vi "Update Enum Getter.vi"(7 "RPC Message Name":string, 8 "error in (no error)":errorcluster, 10 "Message Getter in":refnum<vi>, 11 "RPC Messages Folder (ProjectItem) in":refnum<vi>) -> (0 "error out":errorcluster, 2 "Message Getter out":refnum<vi>, 3 "RPC Messages Folder (ProjectItem) out":refnum<vi>)   [LabVIEW 2019, in "gRPC Template Creation Utility.lvlib"]
uses:
  gRPC Template Creation Utility.lvlib
  <vilib>/Utility/traverseref.llb/VI Scripting - Traverse.lvlib
  <vilib>/Utility/traverseref.llb/TRef TravTarget.ctl
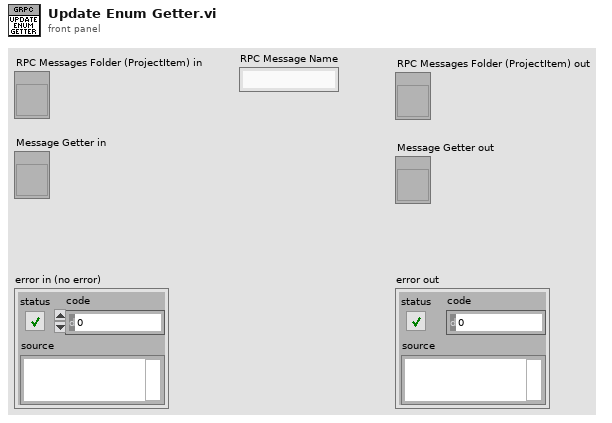
[diagram p1: front panel]
types:
  T1 = typedef "TRef TravTarget.ctl" = enum16{"FP", "BD", "Other"}
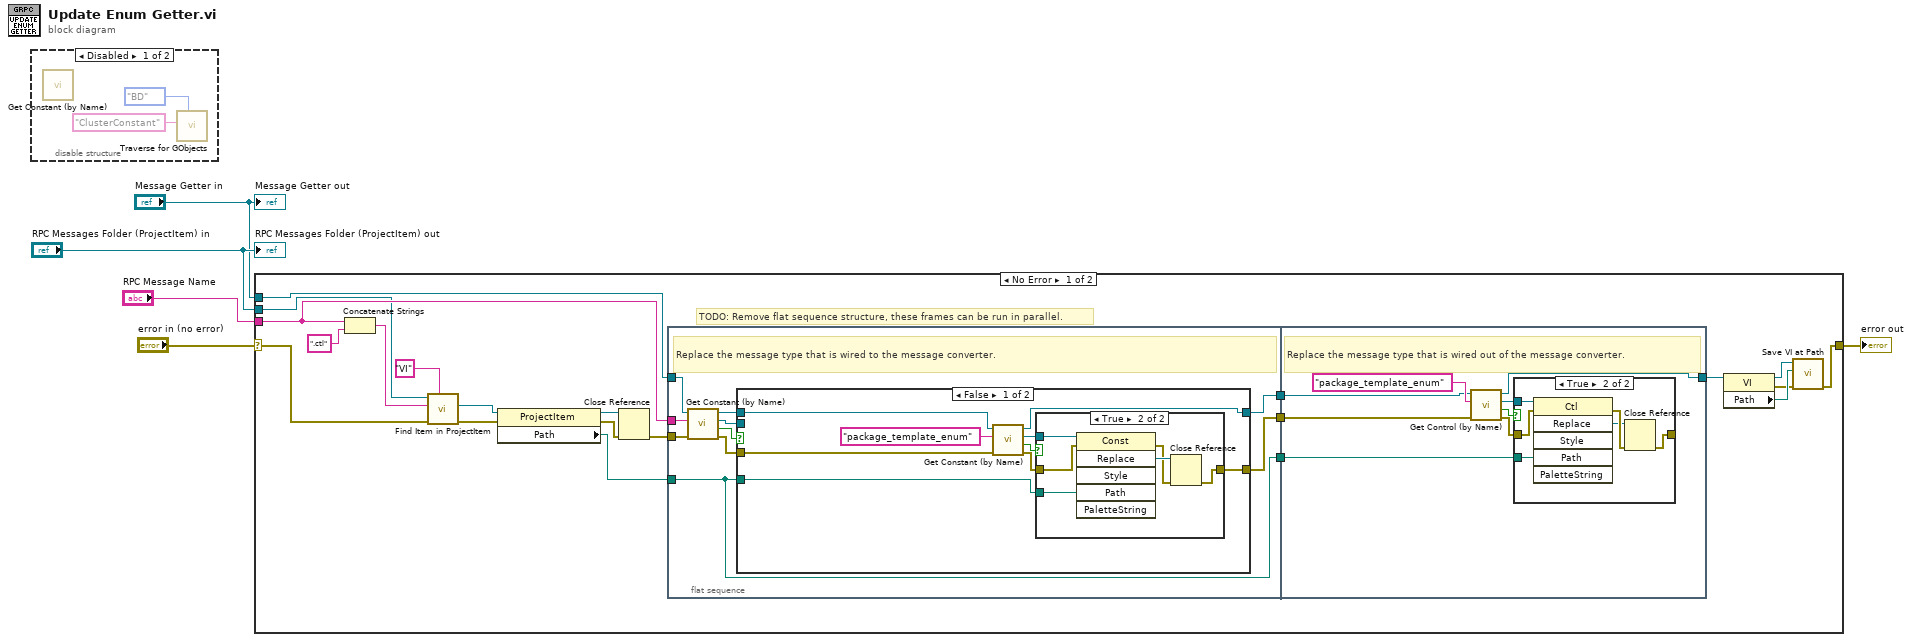
[diagram p0: block diagram]
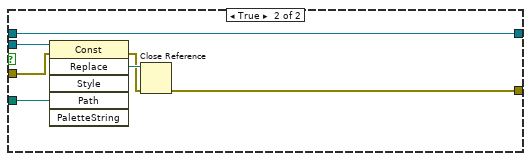
[diagram p4: hidden frame]
diagram:
  n1 = disable-structure shown="Disabled" {
    frame Disabled {
      n2 = call "Get Constant (by Name).vi"() -> ()  [unwired: 8 in, 4 out]
      n3 = call <vilib>:"Traverse for GObjects.vi"("Traverse Target"=TRef_TravTarget."BD", "Class Name"="ClusterConstant") -> ()  [unwired: 6 in, 4 out]
    }
    frame Enabled {
    }
  }
  n4 = case shown="No Error" "error in (no error)" {
    selector: "error in (no error)" -> [w18 w77]
    tunnel: [w16 w77] -> w5
    tunnel: "RPC Message Name" -> [w19 _]
    tunnel: "RPC Messages Folder (ProjectItem) in" -> [w17 _]
    tunnel: "Message Getter in" -> [w14 _]
    frame No Error {
      # "TODO: Remove flat sequence structure, these frames can be run in parallel."
      n5 = Concatenate Strings(w19, ".ctl" ("string")) -> (w22:string)
      n6 = call "Find Item in ProjectItem.vi"("Item Type"="VI", "error in (no error)"=w18, "Name"=w22, "ProjectItem in"=w17) -> ("error out"=w26:errorcluster, "Item Refnum out"=w25:refnum<vi>)  [unwired: 4 in, 2 out]
      n7 = property class="ProjectItem"(reference=w25, error in=w26) -> (reference out=w27:refnum<vi>, error out=w28:errorcluster, "Path"=w20:path)
      n8 = Close Reference(reference=w27, error in (no error)=w28) -> (error out=w15:errorcluster)
      n9 = flat-sequence {
        tunnel: w20 -> [w29]
        tunnel: w15 -> [w37]
        tunnel: w19 -> [w36]
        tunnel: [w38] -> w21
        tunnel: w14 -> [w31]
        tunnel: [w30] -> w10
        tunnel: [w29] -> w9
        tunnel: w21 -> [w65]
        tunnel: w10 -> [w64]
        tunnel: w9 -> [w63]
        tunnel: [w62] -> w8
        frame #0 {
          # "Replace the message type that is wired to the message converter."
          n10 = call "Get Constant (by Name).vi"("error in (no error)"=w37, "Constant Label"=w36, "Owner VI in"=w31) -> ("error out"=w35:errorcluster, "Found ?"=w34:bool, "Const ref out"=w33:refnum<vi>, "Owner VI out"=w32:refnum<vi>)  [unwired: 5 in]
          n11 = case shown="False" w34 {
            tunnel: [w47 w56] -> w38
            tunnel: w29 -> [w46 w57]
            tunnel: w35 -> [w41 w61]
            tunnel: w32 -> [w40 w55]
            tunnel: w33 -> [_ w60]
            tunnel: [w39 w55] -> w30
            frame False {
              n12 = call "Get Constant (by Name).vi"("error in (no error)"=w41, "Constant Label"="package_template_enum" ("name/order"), "Owner VI in"=w40) -> ("error out"=w43:errorcluster, "Found ?"=w42:bool, "Const ref out"=w45:refnum<vi>, "Owner VI out"=w39:refnum<vi>)  [unwired: 5 in]
              n13 = case shown="True" w42 {
                tunnel: [w48 w54] -> w47
                tunnel: w46 -> [_ w53]
                tunnel: w45 -> [_ w50]
                tunnel: w43 -> [w48 w49]
                frame False {
                }
                frame True {
                  n14 = invoke class="Const" method="Replace"(reference=w50, error in=w49, "Path"=w53) -> (error out=w51:errorcluster, "Replace"=w52:refnum<vi>)  [unwired: 3 in, 4 out]
                  n15 = Close Reference(reference=w52, error in (no error)=w51) -> (error out=w54:errorcluster)
                }
              }
            }
            frame True {
              n16 = invoke class="Const" method="Replace"(reference=w60, error in=w61, "Path"=w57) -> (error out=w58:errorcluster, "Replace"=w59:refnum<vi>)  [unwired: 3 in, 4 out]
              n17 = Close Reference(reference=w59, error in (no error)=w58) -> (error out=w56:errorcluster)
            }
          }
        }
        frame #1 {
          # "Replace the message type that is wired out of the message converter."
          n18 = call "Get Control (by Name).vi"("error in (no error)"=w65, "Control Label"="package_template_enum" ("name/order"), "Owner VI in"=w64) -> ("error out"=w69:errorcluster, "Found ?"=w68:bool, "Control Refnum"=w67:refnum<vi>, "Owner VI out"=w62:refnum<vi>)  [unwired: 5 in]
          n19 = case shown="True" w68 {
            tunnel: [w70 w76] -> _
            tunnel: w63 -> [_ w73]
            tunnel: w67 -> [_ w72]
            tunnel: w69 -> [w70 w71]
            frame False {
            }
            frame True {
              n20 = invoke class="Ctl" method="Replace"(reference=w72, error in=w71, "Path"=w73) -> (error out=w75:errorcluster, "Replace"=w74:refnum<vi>)  [unwired: 3 in, 4 out]
              n21 = Close Reference(reference=w74, error in (no error)=w75) -> (error out=w76:errorcluster)
            }
          }
        }
      }
      n22 = property class="VI"(reference=w8) -> (reference out=w12:refnum<vi>, error out=w11:errorcluster, "Path"=w13:path)  [unwired: 1 in]
      n23 = call "Save VI at Path.vi"("error in (no error)"=w11, "Path"=w13, "VI in"=w12) -> ("error out"=w16:errorcluster)  [unwired: 6 in, 2 out]
    }
    frame Error {
    }
  }
  "error out" <- w5
  "RPC Messages Folder (ProjectItem) out" <- "RPC Messages Folder (ProjectItem) in"
  "Message Getter out" <- "Message Getter in"
